vi "FPGA Time Tag.vi"(7 "runs":i32, 8 "error in (no error)":errorcluster, 9 "fileName":string, 10 "fpgaCommand":u8, 11 "saveClicks":bool) -> (0 "error out":errorcluster, 3 "function return":i32, 4 "Stats":i32[](array[numeric]))   [LabVIEW 2012, in "Stats32.lvlib"]
doc: "LIBRARY_API int FPGA_TimeTag(bool saveClicks, unsigned char fpgaCommand,char* fileName, int* stats, int runs);"
uses:
  Stats32.lvlib
  Stats/Release/Win32/Stats32.dll
panel:
  out "fileName out":string
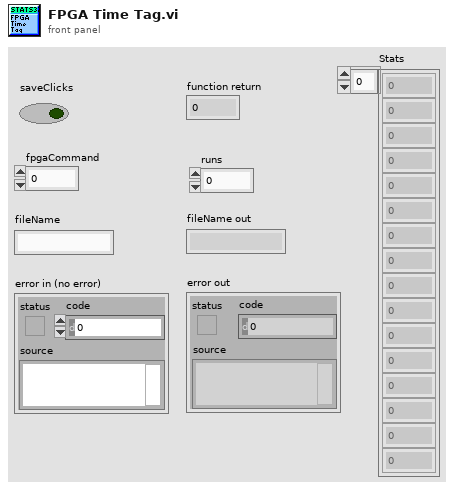
[diagram p1: front panel]
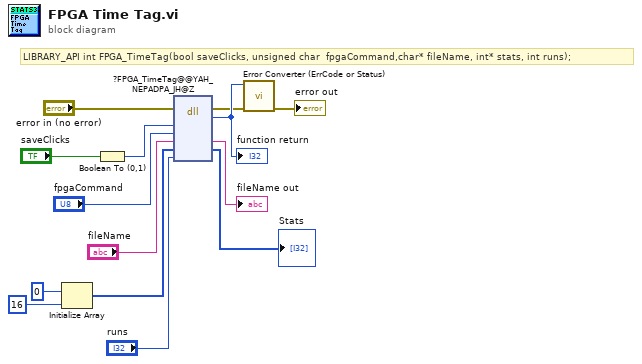
[diagram p0: block diagram]
diagram:
  # "LIBRARY_API int FPGA_TimeTag(bool saveClicks, unsigned char  fpgaCommand,char* fileName, int* stats, int runs);"
  n1 = Initialize Array(0, 16) -> (w1:i32[])
  n2 = Boolean To (0,1)(Boolean="saveClicks") -> (0, 1=w12:i16)
  n3 = dll-call lib="C:/Programming/Stats/Stats/Release/Win32/Stats32.*" fn="?FPGA_TimeTag@@YAH_NEPADPA_JH@Z"(error in="error in (no error)", "saveClicks"=w12, "fpgaCommand"="fpgaCommand", "fileName"="fileName", "stats"=w1, "runs"="runs") -> (error out=w6:errorcluster, "return type"=w14:i32, "fileName"=→"fileName out":string, "stats"=→"Stats":i64[])  [unwired: 5 in, 1 out]
  "function return" <- w14
  n4 = call "Error Converter (ErrCode or Status).vi"("error in (no error)"=w6, "error code"=w14) -> ("error out"=→"error out":errorcluster)  [unwired: 9 in]
